vi "Configure IScan Trigger Mode.vi"(8 "error in (no error)":errorcluster, 10 "IScan Trigger Mode (0: Off)":i32(ring) items=["Off", "Measurement Limit", "Non-monotonic Edge", "Runt", "Serial", "Zone Qualify"], 11 "VISA resource name":refnum<visa-resource-name>) -> (0 "error out":errorcluster, 3 "VISA resource name out":refnum<visa-resource-name>)   [LabVIEW 2020, in "Agilent 90000 Series.lvlib"]
doc: "Selects the type of InfiniiScan trigger mode."
uses:
  Agilent 90000 Series.lvlib
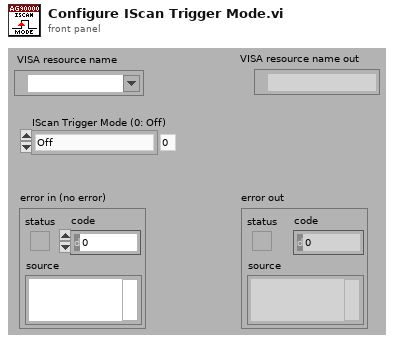
[diagram p1: front panel]
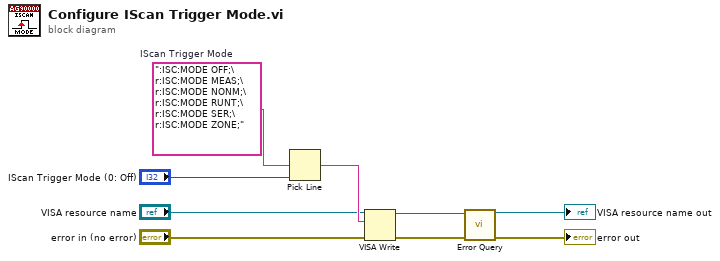
[diagram p0: block diagram]
diagram:
  w9 = ":ISC:MODE OFF;\r:ISC:MODE MEAS;\r:ISC:MODE NONM;\r:ISC:MODE RUNT;\r:ISC:MODE SER;\r:ISC:MODE ZONE;"  # IScan Trigger Mode
  n1 = Pick Line(multi-line string=w9, line index="IScan Trigger Mode (0: Off)") -> (output string=w7:string)  [unwired: 1 out]
  n2 = VISA Write(VISA resource name="VISA resource name", write buffer=w7, error in (no error)="error in (no error)") -> (VISA resource name out=w4:refnum<visa-resource-name>, error out=w3:errorcluster)  [unwired: 1 out]
  n3 = call "Error Query.vi"("error in (no error)"=w3, "VISA resource name"=w4) -> ("error out"=→"error out":errorcluster, "VISA resource name out"=→"VISA resource name out":refnum<visa-resource-name>)  [unwired: 8 out]
